vi "About.vi"() -> ()   [LabVIEW 2018, in "CAN FD.lvlib"]
uses:
  CAN FD.lvlib
panel:
  out "right":string
  out "Version":string
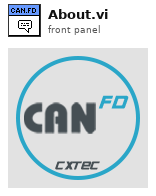
[diagram p1: front panel]
types:
  T1 = enum16{"CharacterArray", "FixedFileInfoCluster", "LanguageCode"}
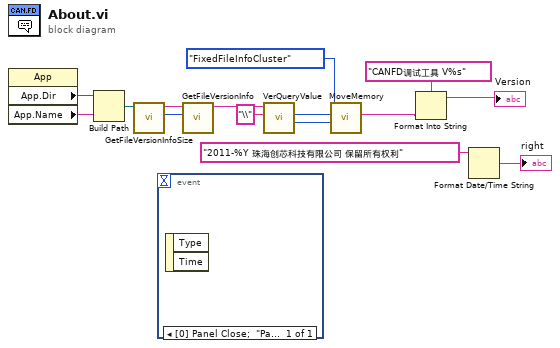
[diagram p0: block diagram]
diagram:
  n1 = property class="App"() -> ("App.Dir"=w12:path, "App.Name"=w13:string)  [unwired: 2 in, 2 out]
  n2 = Build Path(base path=w12, name or relative path=w13) -> (appended path=w11:path)
  n3 = call <vilib>:"GetFileVersionInfoSize.vi"("Path"=w11) -> ("Size"=w14:i32, "lptstrFilename"=w15:string)  [unwired: 8 in, 1 out]
  n4 = event shown="[0] Panel Close;  \"Pane\": Mouse Up" {
    selector: _ -> [_]
    dyn-events: _ -> [_]
    timeout: _ -> [_]
    event Panel Close; Mouse Up {
      n5 = event-data() -> ()  [unwired: 1 in, 2 out]
    }
  }
  n6 = call <vilib>:"GetFileVersionInfo.vi"("Size"=w14, "lptstrFilename"=w15) -> ("lpData"=w10:string)  [unwired: 8 in, 1 out]
  n7 = call <vilib>:"VerQueryValue.vi"("lpSubBlock"="\\", "lpData"=w10) -> ("puLen"=w7:u32, "lplpBuffer"=w8:u64)  [unwired: 7 in, 1 out]
  n8 = call <vilib>:"MoveMemory.vi"("puLen"=w7, "lplpBuffer"=w8, "Datatype"=T1."FixedFileInfoCluster") -> ("data"=w5:string)  [unwired: 7 in, 1 out]
  n9 = Format Into String(format string="CANFD调试工具 V%s", w5) -> (resulting string=→"Version":string)  [unwired: 2 in, 1 out]
  n10 = Format Date/Time String(time format string (%c)="2011-%Y 珠海创芯科技有限公司 保留所有权利") -> (date/time string=→"right":string)  [unwired: 2 in]
